vi "Auto - Increment State (SubVI).vi"(6 "numberOfBallsShot out":dbl, 7 "Was Disabled":bool, 8 "Constant cluster In":T2, 9 "Auton Cluster In":T3, 10 "Sensors In":T1, 11 "Auton State In":i32) -> (0 "Constant cluster Out":T2, 1 "Auton cluster Out":T3, 2 "Sensors Out":T1, 3 "Auton State Out":i32, 4 "End Condition":dbl)   [LabVIEW 2020]
uses:
  TypeDefs/Auton Cluster Typedef.ctl
  Disabled/Constant VI_s/Disabled - Constant Cluster Typedef.ctl
  TypeDefs/Sensor TypeDef.ctl
panel:
  out "Distance Driven":dbl
  out "Dist to Drive":dbl
  # "Inputs"
  # "Outputs"
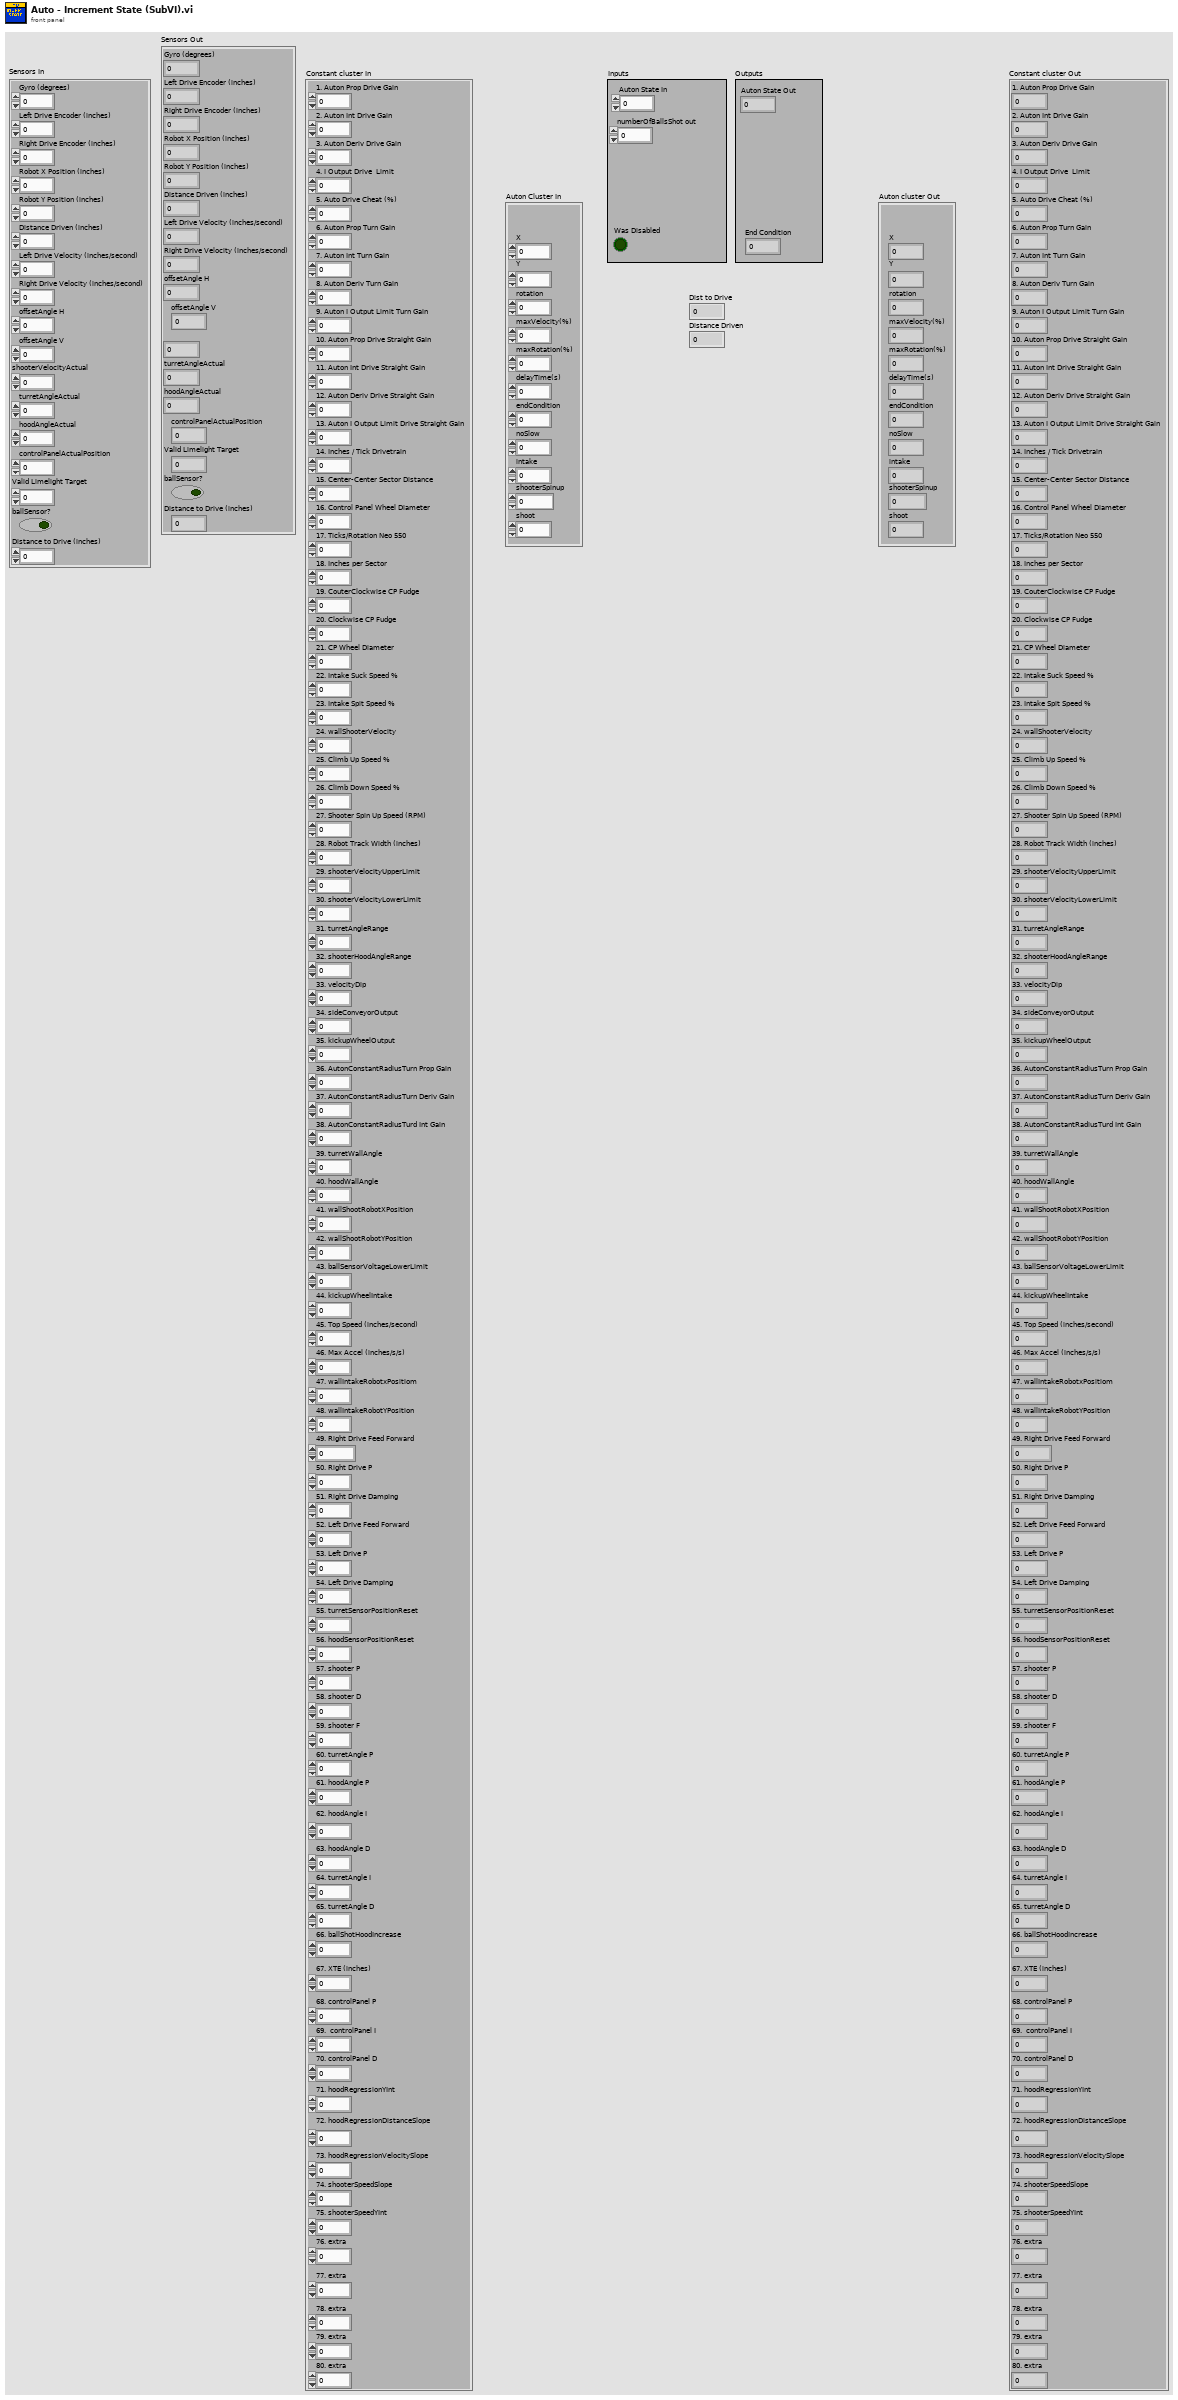
[diagram p1: front panel]
types:
  T1 = typedef "Sensor TypeDef.ctl" = cluster{"Gyro (degrees)":dbl, "Left Drive Encoder (inches)":dbl, "Right Drive Encoder (inches)":dbl, "Robot X Position (inches)":dbl, "Robot Y Position (inches)":dbl, "Distance Driven (inches)":dbl, "Left Drive Velocity (inches/second)":dbl, "Right Drive Velocity (inches/second)":dbl, "offsetAngle H":dbl, "offsetAngle V":dbl, "shooterVelocityActual":dbl, "turretAngleActual":dbl, "hoodAngleActual":dbl, "controlPanelActualPosition":dbl, "Valid Limelight Target":dbl, "ballSensor?":bool, "Distance to Drive (inches)":dbl}
  T2 = typedef "Disabled - Constant Cluster Typedef.ctl" = cluster{"1. Auton Prop Drive Gain":dbl, "2. Auton Int Drive Gain":dbl, "3. Auton Deriv Drive Gain":dbl, "4. I Output Drive  Limit":dbl, "5. Auto Drive Cheat (%)":dbl, "6. Auton Prop Turn Gain":dbl, "7. Auton Int Turn Gain":dbl, "8. Auton Deriv Turn Gain":dbl, "9. Auton I Output Limit Turn Gain":dbl, "10. Auton Prop Drive Straight Gain":dbl, "11. Auton Int Drive Straight Gain":dbl, "12. Auton Deriv Drive Straight Gain":dbl, "13. Auton I Output Limit Drive Straight Gain":dbl, "14. Inches / Tick Drivetrain":dbl, "15. Center-Center Sector Distance":dbl, "16. Control Panel Wheel Diameter":dbl, "17. Ticks/Rotation Neo 550":dbl, "18. Inches per Sector":dbl, "19. CouterClockwise CP Fudge":dbl, "20. Clockwise CP Fudge":dbl, "21. CP Wheel Diameter":dbl, "22. Intake Suck Speed %":dbl, "23. Intake Spit Speed %":dbl, "24. wallShooterVelocity":dbl, "25. Climb Up Speed %":dbl, "26. Climb Down Speed %":dbl, "27. Shooter Spin Up Speed (RPM)":dbl, "28. Robot Track Width (inches)":dbl, "29. shooterVelocityUpperLimit":dbl, "30. shooterVelocityLowerLimit":dbl, "31. turretAngleRange":dbl, "32. shooterHoodAngleRange":dbl, "33. velocityDip":dbl, "34. sideConveyorOutput":dbl, "35. kickupWheelOutput":dbl, "36. AutonConstantRadiusTurn Prop Gain":dbl, "37. AutonConstantRadiusTurn Deriv Gain":dbl, "38. AutonConstantRadiusTurd Int Gain":dbl, "39. turretWallAngle":dbl, "40. hoodWallAngle":dbl, "41. wallShootRobotXPosition":dbl, "42. wallShootRobotYPosition":dbl, "43. ballSensorVoltageLowerLimit":dbl, "44. kickupWheelIntake":dbl, "45. Top Speed (inches/second)":dbl, "46. Max Accel (inches/s/s)":dbl, "47. wallIntakeRobotxPositiom":dbl, "48. wallIntakeRobotYPosition":dbl, "49. Right Drive Feed Forward":dbl, "50. Right Drive P":dbl, "51. Right Drive Damping":dbl, "52. Left Drive Feed Forward":dbl, "53. Left Drive P":dbl, "54. Left Drive Damping":dbl, "55. turretSensorPositionReset":dbl, "56. hoodSensorPositionReset":dbl, "57. shooter P":dbl, "58. shooter D":dbl, "59. shooter F":dbl, "60. turretAngle P":dbl, "61. hoodAngle P":dbl, "62. hoodAngle I":dbl, "63. hoodAngle D":dbl, "64. turretAngle I":dbl, "65. turretAngle D":dbl, "66. ballShotHoodIncrease":dbl, "67. XTE (inches)":dbl, "68. controlPanel P":dbl, "69.  controlPanel I":dbl, "70. controlPanel D":dbl, "71. hoodRegressionYInt":dbl, "72. hoodRegressionDistanceSlope":dbl, "73. hoodRegressionVelocitySlope":dbl, "74. shooterSpeedSlope":dbl, "75. shooterSpeedYInt":dbl, "76. extra":dbl, "77. extra":dbl, "78. extra":dbl, "79. extra":dbl, "80. extra":dbl}
  T3 = typedef "Auton Cluster Typedef.ctl" = cluster{"rotation":dbl, "maxVelocity(%)":dbl, "delayTime(s)":dbl, "endCondition":dbl, "noSlow":dbl, "intake":dbl, "shooterSpinup":dbl, "shoot":dbl, "X":dbl, "Y":dbl, "maxRotation(%)":dbl}
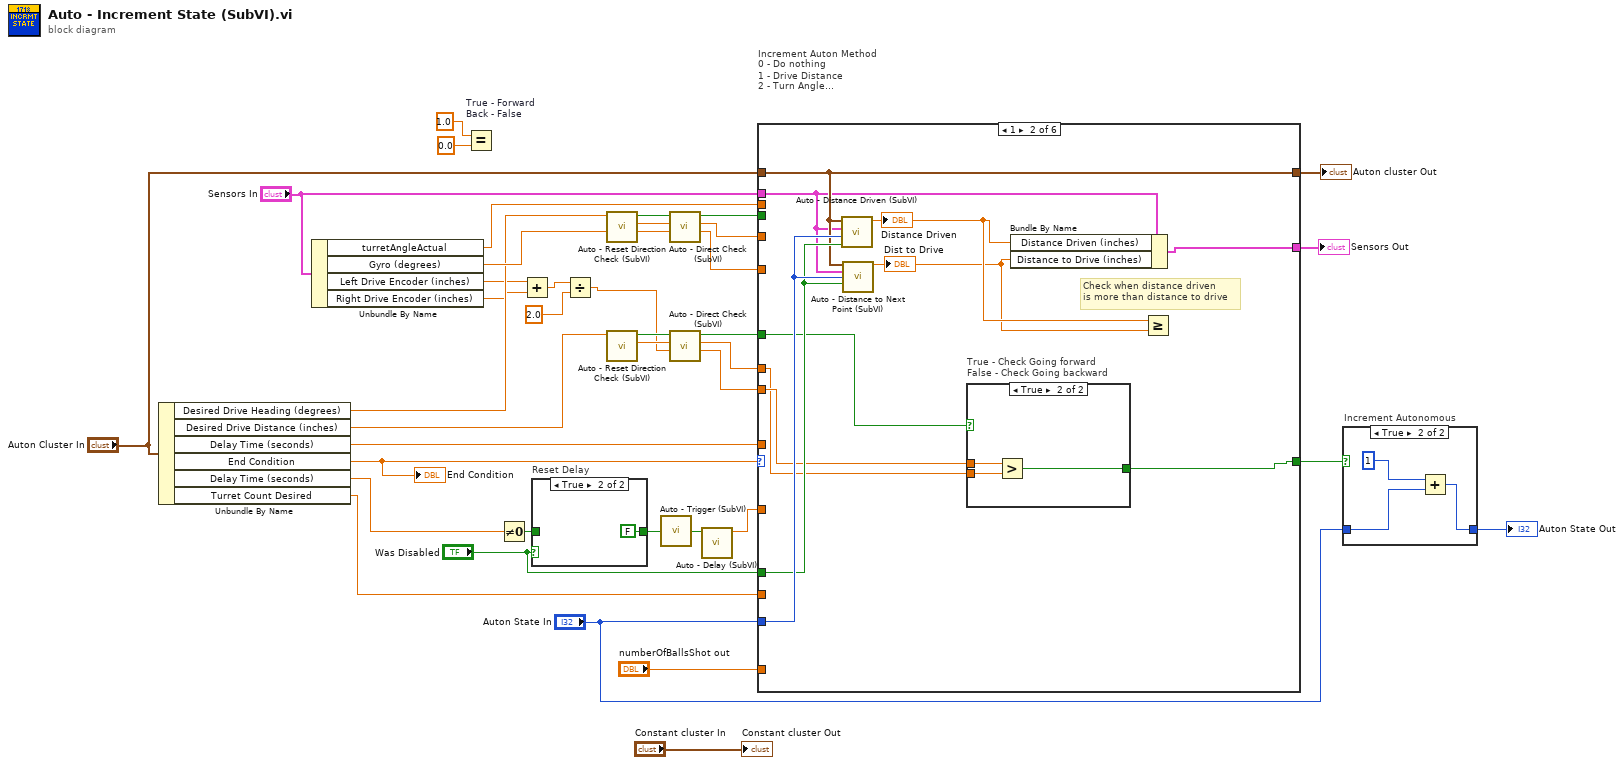
[diagram p0: block diagram]
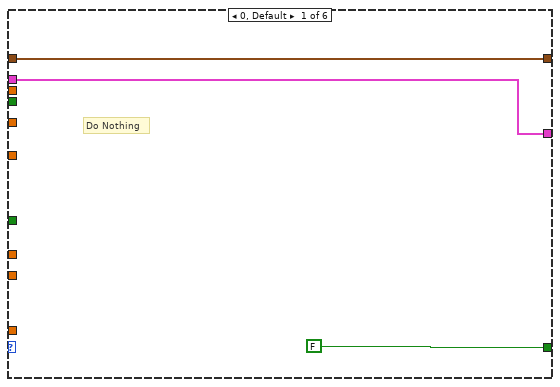
[diagram p4: hidden frame]
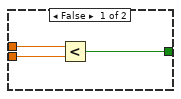
[diagram p5: hidden frame]
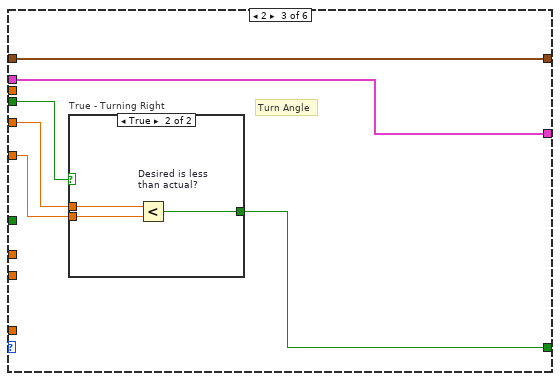
[diagram p6: hidden frame]
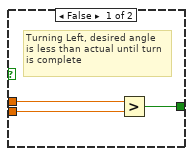
[diagram p7: hidden frame]
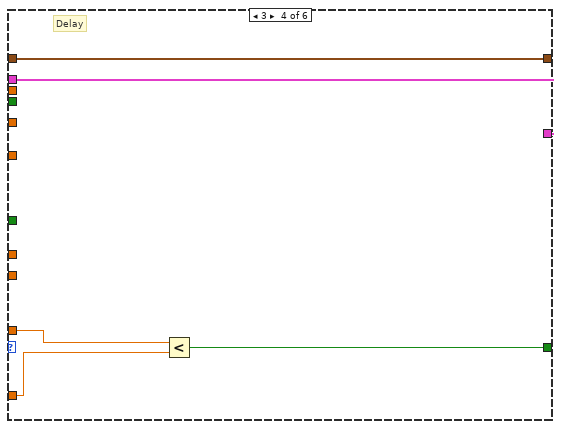
[diagram p8: hidden frame]
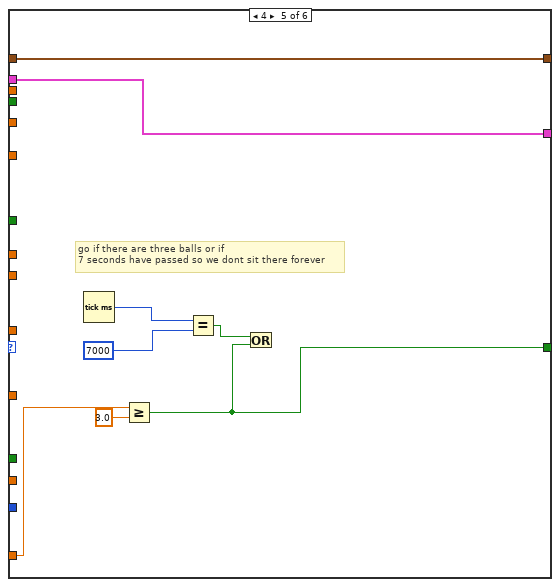
[diagram p9: hidden frame]
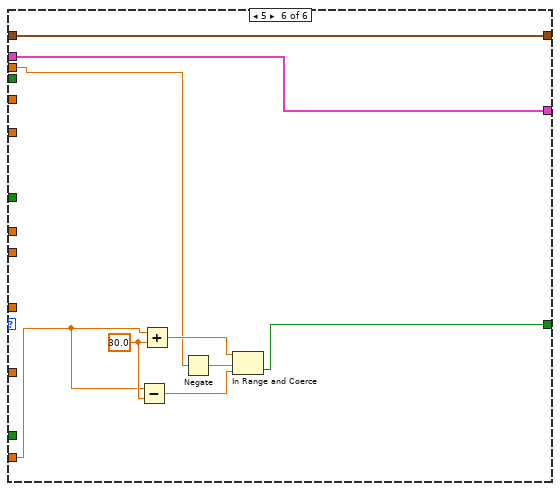
[diagram p10: hidden frame]
diagram:
  n1 = Unbundle By Name("Auton Cluster In") -> ("Desired Drive Heading (degrees)"=w17:dbl, "Desired Drive Distance (inches)"=w2:dbl, "Delay Time (seconds)"=w35:dbl, "End Condition"=w22:dbl, "Delay Time (seconds)"=w30:dbl, "Turret Count Desired"=w3:dbl)
  "End Condition" <- w22
  n2 = Unbundle By Name("Sensors In") -> ("turretAngleActual"=w4:dbl, "Gyro (degrees)"=w23:dbl, "Left Drive Encoder (inches)"=w14:dbl, "Right Drive Encoder (inches)"=w13:dbl)
  n3 = Equal? "True - Forward\nBack - False"(x=1.0, y=0.0) -> ()  [unwired: 1 out]
  n4 = Not Equal To 0?(x=w30) -> (x != 0?=w28:bool)
  n5 = Add(x=w14, y=w13) -> (x+y=w12:dbl)
  n6 = case "Reset Delay" shown="True" "Was Disabled" {
    tunnel: [w40 FALSE] -> w27
    tunnel: w28 -> [w40 _]
    frame False {
    }
    frame True {
    }
  }
  n7 = Divide(x=w12, y=2.0) -> (x/y=w8:dbl)
  n8 = call "Auto - Reset Direction Check (SubVI).vi"("Desired In"=w17) -> ("Desired out"=w33:dbl, "Reset Direction"=w32:bool)  [unwired: 9 in]
  n9 = call "Auto - Reset Direction Check (SubVI).vi"("Desired In"=w2) -> ("Desired out"=w9:dbl, "Reset Direction"=w10:bool)  [unwired: 9 in]
  n10 = call "Auto - Trigger (SubVI).vi"("Trigger"=w27) -> ("Trigger Output"=w31:bool)
  n11 = call "Auto - Direct Check (SubVI).vi"("Process Variable In"=w23, "Set Point In"=w33, "Trigger Output"=w32) -> ("Process Variable Out"=w36:dbl, "Set Point Out"=w37:dbl, "True - Going Forward"=w34:bool)  [unwired: 6 in]
  n12 = call "Auto - Direct Check (SubVI).vi"("Process Variable In"=w8, "Set Point In"=w9, "Trigger Output"=w10) -> ("Process Variable Out"=w6:dbl, "Set Point Out"=w1:dbl, "True - Going Forward"=w7:bool)  [unwired: 6 in]
  n13 = call "Auto - Delay (SubVI).vi"("Trigger Input"=w31) -> ("Elapsed Time (seconds)"=w29:dbl)  [unwired: 10 in]
  n14 = case "Increment Auton Method\n0 - Do nothing\n1 - Drive Distance\n2 - Turn Angle\n3 - Delay (seconds)\n4 - Number of balls fired (3)\n5 - Turn Turret to Angle" shown="1" w22 {
    tunnel: [FALSE ("Time Expired") w45 w66 w76 w79 w91] -> w38
    tunnel: w36 -> [_ _ w67 _ _ _]
    tunnel: w37 -> [_ _ w64 _ _ _]
    tunnel: w35 -> [_ _ _ w78 _ _]
    tunnel: w34 -> [_ _ w65 _ _ _]
    tunnel: w29 -> [_ _ _ w77 _ _]
    tunnel: "Auton Cluster In" -> [w43 w53 w63 w75 w84 w90]
    tunnel: [w43 w53 w63 w75 w84 w90] -> w24
    tunnel: "Auton State In" -> [_ w55 _ _ _ _]
    tunnel: "Was Disabled" -> [_ w54 _ _ _ _]
    tunnel: "Sensors In" -> [w42 w52 w62 w74 w83 w89]
    tunnel: [w42 w49 w62 w74 w83 w89] -> w16
    tunnel: w7 -> [_ w48 _ _ _ _]
    tunnel: w6 -> [_ w47 _ _ _ _]
    tunnel: w1 -> [_ w46 _ _ _ _]
    tunnel: "numberOfBallsShot out" -> [_ _ _ _ w86 _]
    tunnel: w4 -> [_ _ _ _ _ w87]
    tunnel: w3 -> [_ _ _ _ _ w94]
    frame 0, Default {
      # "Do Nothing"
    }
    frame 1 {
      # "Check when distance driven\nis more than distance to drive"
      n15 = call "Auto - Distance Driven (SubVI).vi"("Was Disabled"=w54, "Auton State In"=w55, "Sensors In"=w52, "Auton Cluster In"=w53) -> ("Distance Driven"=w51:dbl)  [unwired: 7 in]
      "Distance Driven" <- w51
      n16 = call "Auto - Distance to Next Point (SubVI).vi"("Auton Cluster In"=w53, "Sensors In"=w52, "Auton State In"=w55, "Was Disabled"=w54) -> ("Distance to Next Point"=w50:dbl)  [unwired: 11 in]
      "Dist to Drive" <- w50
      n17 = case "True - Check Going forward\nFalse - Check Going backward" shown="True" w48 {
        tunnel: w47 -> [w58 w61]
        tunnel: w46 -> [w57 w60]
        tunnel: [w56 w59] -> w45
        frame False {
          n18 = Less?(x=w58, y=w57) -> (x < y?=w56:bool)
        }
        frame True {
          n19 = Greater?(x=w61, y=w60) -> (0:w59:bool)
        }
      }
      n20 = Bundle By Name(cluster=w52, "Distance Driven (inches)"=w51, "Distance to Drive (inches)"=w50) -> (w49:T1)
      n21 = Greater Or Equal?(x=w51, y=w50) -> ()  [unwired: 1 out]
    }
    frame 2 {
      # "Turn Angle"
      n22 = case "True - Turning Right" shown="True" w65 {
        tunnel: [w69 w73] -> w66
        tunnel: w67 -> [w70 w72]
        tunnel: w64 -> [w68 w71]
        frame False {
          # "Turning Left, desired angle\nis less than actual until turn\nis complete"
          n23 = Greater?(x=w68, y=w70) -> (0:w69:bool)
        }
        frame True {
          n24 = Less? "Desired is less\nthan actual?"(x=w71, y=w72) -> (x < y?=w73:bool)
        }
      }
    }
    frame 3 {
      # "Delay"
      n25 = Less?(x=w78, y=w77) -> (x < y?=w76:bool)
    }
    frame 4 {
      # "go if there are three balls or if \n7 seconds have passed so we dont sit there forever"
      n26 = Tick Count (ms)() -> (millisecond timer value=w82:u32)
      n27 = Greater Or Equal?(x=w86, y=3.0) -> (x >= y?=w79:bool)
      n28 = Equal?(x=w82, y=u32 7000) -> (x = y?=w80:bool)
      n29 = Or(x=w80, y=w79) -> ()  [unwired: 1 out]
    }
    frame 5 {
      w95 = 30.0 ("y")
      n30 = Subtract(x=w94, y=w95) -> (x-y=w92:dbl)
      n31 = Add(x=w94, y=w95) -> (x+y=w93:dbl)
      n32 = Negate(x=w87) -> (-x=w88:dbl)
      n33 = In Range and Coerce(upper limit=w93, x=w88, lower limit=w92) -> (In Range?=w91:bool)  [unwired: 1 out]
    }
  }
  "Auton cluster Out" <- w24
  "Sensors Out" <- w16
  n34 = case "Increment Autonomous" shown="True" w38 {
    tunnel: "Auton State In" -> [w96 w98]
    tunnel: [w96 w99] -> w39
    frame False {
    }
    frame True {
      n35 = Add(x=1, y=w98) -> (x+y=w99:i32)
    }
  }
  "Auton State Out" <- w39
  "Constant cluster Out" <- "Constant cluster In"
